vi "Drive Check for New Command.vi"(9 "input cluster":T6, 10 "Wait time (ms)":dbl, 11 "Finished?":bool) -> (0 "Completion":T4, 1 "Subsystem Name":string, 2 "SetPoint":T1, 3 "Initial Trace String":string, 4 "output cluster":T6)   [LabVIEW 2015]
doc: "This VI is called for each controller loop iteration. It checks for new commands, updates timing data, and upon completion, notifies and waiting commands."
uses:
  Drive Setpoints.ctl
  Drive Operations.ctl
  <vilib>/Rock Robotics/WPI/Framework/Command Status Info.ctl
  <vilib>/Rock Robotics/WPI/Framework/Completion Status.ctl
  <vilib>/Rock Robotics/WPI/Framework/Completion Notifier.ctl
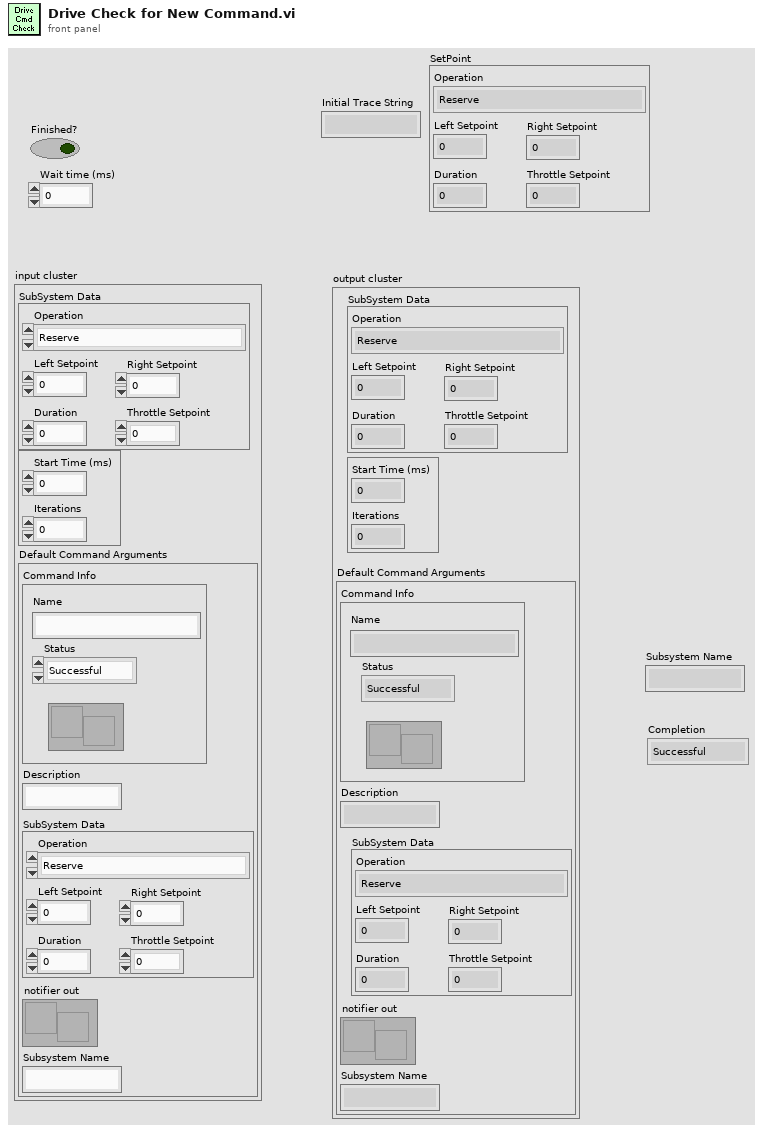
[diagram p1: front panel]
types:
  T1 = typedef "Drive Setpoints.ctl" = cluster{"Operation":T2, "Left Setpoint":dbl, "Right Setpoint":dbl, "Duration":dbl, "Throttle Setpoint":dbl}
  T2 = typedef "Drive Operations.ctl" = enum16{"Reserve", "Read Current", "Immediate", "Drive for Time", "Drive for Distance"}
  T3 = typedef "Command Status Info.ctl" = cluster{"Name":string, "Status":T4, "notifier out":T5}
  T4 = typedef "Completion Status.ctl" = enum16{"Successful", "Aborted", "Incomplete"}
  T5 = typedef "Completion Notifier.ctl" = refnum<notifier>
  T6 = cluster{"SubSystem Data":T1, cluster{"Start Time (ms)":u32, "Iterations":i32}, "Default Command Arguments":cluster{"Command Info":T3, "Description":string, "SubSystem Data":T1, "notifier out":refnum<notifier>, "Subsystem Name":string}}
  T7 = cluster{"Command Info":T3, "Description":string, "SubSystem Data":T1, "notifier out":refnum<notifier>, "Subsystem Name":string}
  T8 = cluster{"SubSystem Data":T1, "Command Info":T3, "Description":string}
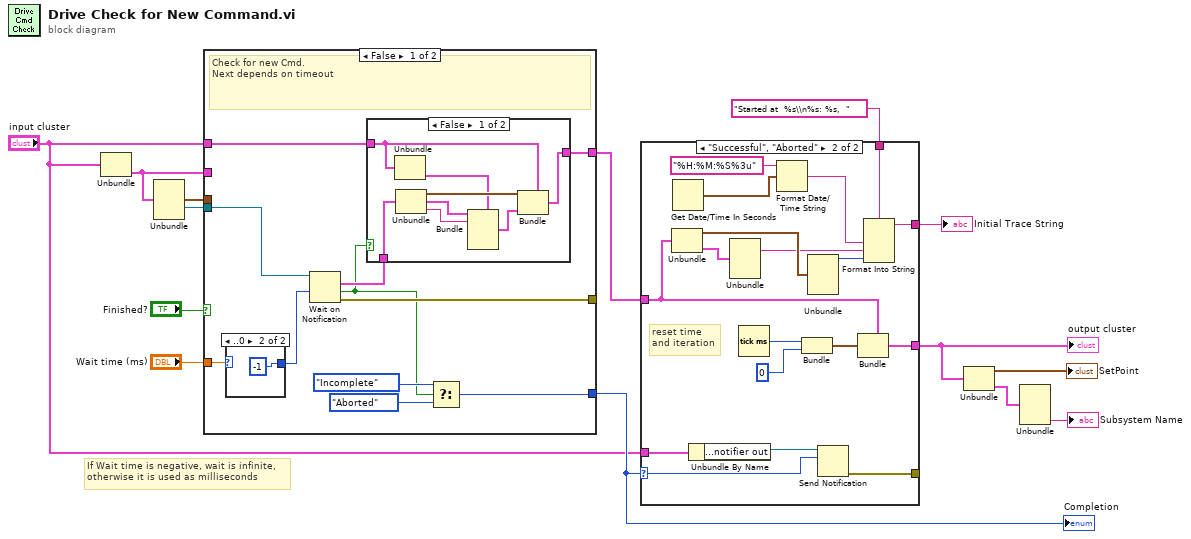
[diagram p0: block diagram]
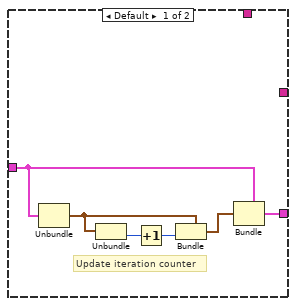
[diagram p2: hidden frame]
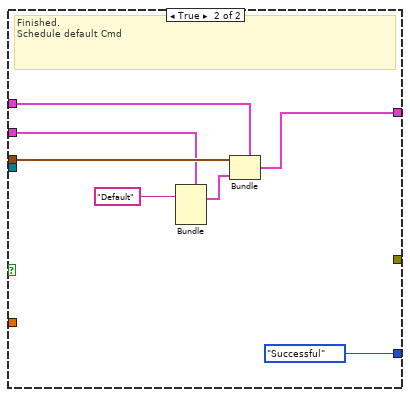
[diagram p5: hidden frame]
diagram:
  # "If Wait time is negative, wait is infinite,\notherwise it is used as milliseconds"
  n1 = Unbundle("input cluster") -> ("Default Command Arguments"=w1:T7)  [unwired: 2 out]
  n2 = Unbundle(w1) -> ("SubSystem Data"=w4:T1, "notifier out"=w5:refnum<notifier>)  [unwired: 3 out]
  n3 = case shown="False" "Finished?" {
    tunnel: [w15 w42] -> w10
    tunnel: "Wait time (ms)" -> [w20 _]
    tunnel: [w23 Completion_Status."Successful"] -> w14
    tunnel: [w25 _] -> _
    tunnel: w5 -> [w24 _]
    tunnel: "input cluster" -> [w17 w41]
    tunnel: w4 -> [_ w40]
    tunnel: w1 -> [_ w38]
    frame False {
      # "Check for new Cmd.\nNext depends on timeout"
      n4 = case shown="..0" w20 {
        selector: w20 -> [w35 _]
        tunnel: [w35 -1] -> w19
        frame Default {
        }
        frame ..0 {
        }
      }
      n5 = Wait on Notification(notifier=w24, timeout in ms (-1)=w19) -> (notification=w18:T8, timed out?=w16:bool, error out=w25:errorcluster)  [unwired: 2 in, 1 out]
      n6 = case shown="False" w16 {
        tunnel: w18 -> [w33 _]
        tunnel: w17 -> [w30 w34]
        tunnel: [w26 w34] -> w15
        frame False {
          n7 = Unbundle(w30) -> ("Default Command Arguments"=w29:T7)  [unwired: 2 out]
          n8 = Unbundle(w33) -> ("SubSystem Data"=w32:T1, "Command Info"=w27:T3, "Description"=w28:string)
          n9 = Bundle(cluster=w29, "Command Info"=w27, "Description"=w28) -> (w31:T7)  [unwired: 3 in]
          n10 = Bundle(cluster=w30, "SubSystem Data"=w32, "Default Command Arguments"=w31) -> (w26:T6)  [unwired: 1 in]
        }
        frame True {
        }
      }
      n11 = Select(t=Completion_Status."Incomplete", s=w16, f=Completion_Status."Aborted") -> (s? t:f=w23:T4)
    }
    frame True {
      # "Finished.\nSchedule default Cmd"
      n12 = Bundle(cluster=w38, "Description"="Default") -> (w39:T7)  [unwired: 4 in]
      n13 = Bundle(cluster=w41, "SubSystem Data"=w40, "Default Command Arguments"=w39) -> (w42:T6)  [unwired: 1 in]
    }
  }
  "Completion" <- w14
  n14 = case shown="\"Successful\", \"Aborted\"" w14 {
    selector: w14 -> [_ w67]
    tunnel: "input cluster" -> [_ w55]
    tunnel: "Started at  %s\\n%s: %s,  " ("format string") -> [_ w64]
    tunnel: [_ w63] -> w12
    tunnel: w10 -> [w46 w56]
    tunnel: [w47 w60] -> w9
    tunnel: [_ w57] -> _
    frame Default {
      # "Update iteration counter"
      n15 = Unbundle(w46) -> (w45:cluster{"Start Time (ms)":u32, "Iterations":i32})  [unwired: 2 out]
      n16 = Unbundle(w45) -> ("Iterations"=w48:i32)  [unwired: 1 out]
      n17 = Increment(x=w48) -> (x+1=w49:i32)
      n18 = Bundle(cluster=w45, "Iterations"=w49) -> (w44:cluster{"Start Time (ms)":u32, "Iterations":i32})  [unwired: 1 in]
      n19 = Bundle(cluster=w46, w44) -> (w47:T6)  [unwired: 2 in]
    }
    frame "Successful", "Aborted" {
      # "reset time\nand iteration"
      n20 = Unbundle(w56) -> ("SubSystem Data"=w62:T1, "Default Command Arguments"=w58:T7)  [unwired: 1 out]
      n21 = Get Date/Time In Seconds() -> (seconds since 1Jan1904=w51:timestamp)
      n22 = Unbundle By Name(w55) -> ("Default Command Arguments.Command Info.notifier out"=w66:T5)
      n23 = Unbundle(w58) -> ("Description"=w53:string)  [unwired: 4 out]
      n24 = Tick Count (ms)() -> (millisecond timer value=w54:u32)
      n25 = Format Date/Time String(time format string (%c)="%H:%M:%S%3u", seconds (now)=w51) -> (date/time string=w50:string)  [unwired: 1 in]
      n26 = Bundle("millisecond timer value"=w54, 0) -> (w59:cluster{"millisecond timer value":u32, i32})  [unwired: 1 in]
      n27 = Unbundle(w62) -> ("Operation"=w65:T2)  [unwired: 4 out]
      n28 = Send Notification(notification=w67, notifier=w66) -> (error out=w57:errorcluster)  [unwired: 1 in, 1 out]
      n29 = Bundle(cluster=w56, w59) -> (w60:T6)  [unwired: 2 in]
      n30 = Format Into String(format string=w64, w50, w53, w65) -> (resulting string=w63:string)  [unwired: 2 in, 1 out]
    }
  }
  "output cluster" <- w9
  "Initial Trace String" <- w12
  n31 = Unbundle(w9) -> ("SubSystem Data"=→"SetPoint":T1, "Default Command Arguments"=w3:T7)  [unwired: 1 out]
  n32 = Unbundle(w3) -> ("Subsystem Name"=→"Subsystem Name":string)  [unwired: 4 out]
